vi "MOVIE_calculate_acquisition_Progress.vi"(4 "error in":errorcluster, 7 "N frames":i32=25) -> (0 "error out":errorcluster, 1 "Slider save movie":u8(slide) scale=0.0..100.0, 2 "kinetic time (s)":sgl, 3 "N frames acquired":i32=25)   [LabVIEW 2015]
uses:
  GLOBAL/Global_CAMERA.vi
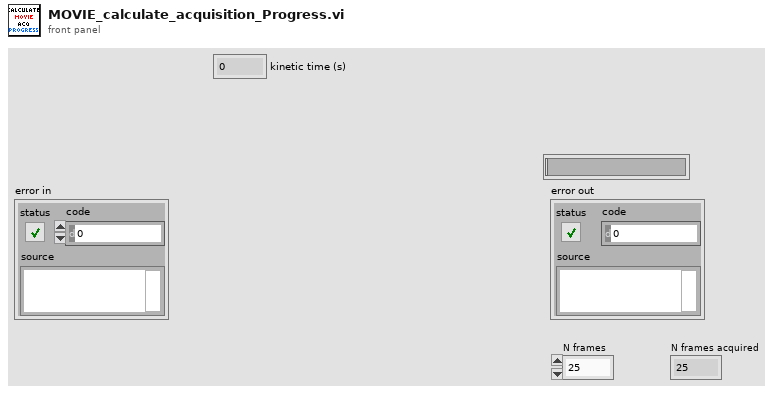
[diagram p1: front panel]
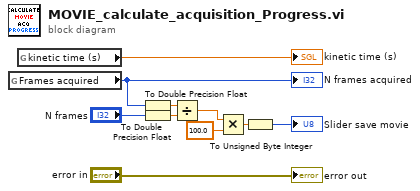
[diagram p0: block diagram]
diagram:
  n1 = global read "Global_CAMERA.vi" "Frames acquired"() -> (w4:i32)
  "N frames acquired" <- w4
  n2 = global read "Global_CAMERA.vi" "kinetic time (s)"() -> (→"kinetic time (s)":sgl)
  n3 = To Double Precision Float(number=w4) -> (double precision float=w8:dbl)
  n4 = To Double Precision Float(number="N frames") -> (double precision float=w9:dbl)
  n5 = Divide(x=w8, y=w9) -> (x/y=w7:dbl)
  n6 = Multiply(x=w7, y=100.0) -> (x*y=w5:dbl)
  n7 = To Unsigned Byte Integer(number=w5) -> (unsigned 8bit integer=→"Slider save movie":u8)
  "error out" <- "error in"
